vi "Init.vi"(7 "Attributes (HttpOnly)":T1={"Expires"=timestamp(0 s since 1904-01-01), "Secure"=FALSE, "HttpOnly"=TRUE, "Domain"="", "Path"="", "SameSite"=enum."Unset (Lax)", "Prefix"=enum."None", "Max-Age Expiry"=TRUE}, 8 "error in (no error)":errorcluster, 10 "Value":string, 11 "Name":string) -> (0 "error out":errorcluster, 3 "Cookie out":refnum<class "Cookie.lvclass">)   [LabVIEW 2020, in "HTTP Utils.lvlib" / "Cookie.lvclass"]
uses:
  Cookie.lvclass
  Cookie Attributes.ctl
  Cookie SameSite.ctl
  Cookie Prefix.ctl
  Cookie.lvclass/Cookie.ctl
  HTTP Utils.lvlib
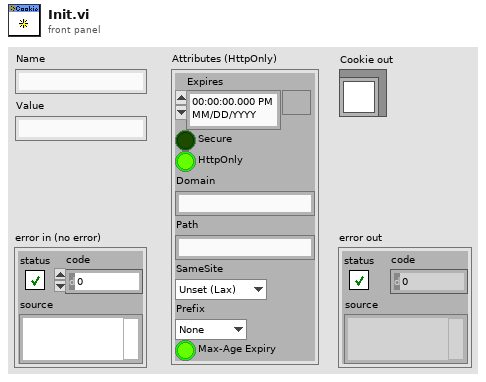
[diagram p1: front panel]
types:
  T1 = typedef "HTTP Utils.lvlib/Cookie Attributes.ctl" = cluster{"Expires":timestamp, "Secure":bool, "HttpOnly":bool, "Domain":string, "Path":string, "SameSite":T2, "Prefix":T3, "Max-Age Expiry":bool}
  T2 = typedef "HTTP Utils.lvlib/Cookie SameSite.ctl" = enum16{"Unset (Lax)", "Lax", "Strict", "None"}
  T3 = typedef "HTTP Utils.lvlib/Cookie Prefix.ctl" = enum16{"None", "Host", "Secure"}
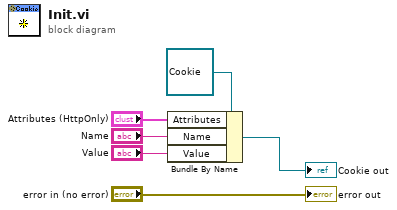
[diagram p0: block diagram]
diagram:
  n1 = Bundle By Name(cluster=refnum<class "Cookie.lvclass"> refnum ("Cookie in"), "Attributes"="Attributes (HttpOnly)", "Name"="Name", "Value"="Value") -> (→"Cookie out":refnum<class "Cookie.lvclass">)
  "error out" <- "error in (no error)"
